vi "Test_OpenCloseTableRef_NoError.vi"(8 "error in (no error)":errorcluster, 11 "TestCase in":refnum<class "TestTopicLookupTable.lvclass">) -> (0 "error out":errorcluster, 3 "TestCase out":refnum<class "TestTopicLookupTable.lvclass">)   [LabVIEW 2017, in "TestTopicLookupTable.lvclass"]
uses:
  TestTopicLookupTable.lvclass
  Source/Mediator/TopicLookupTable/TopicLookupTable.lvclass
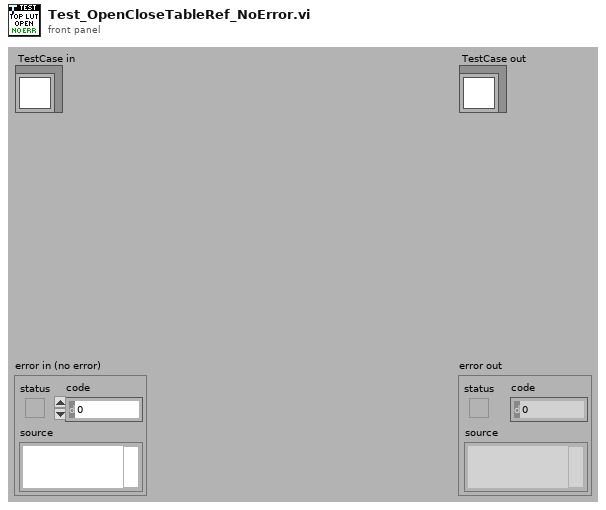
[diagram p1: front panel]
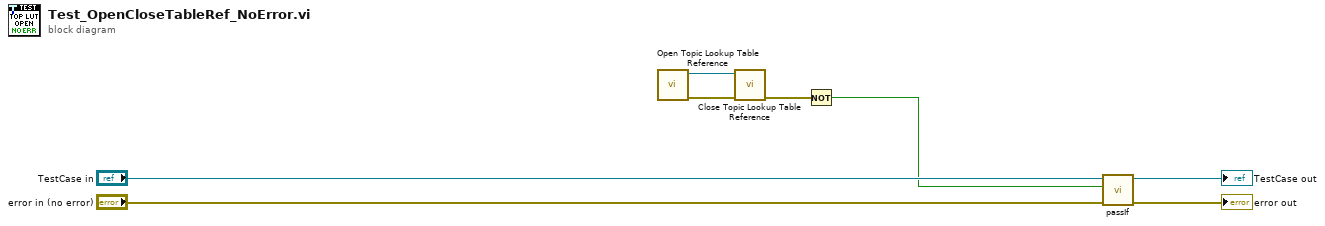
[diagram p0: block diagram]
diagram:
  n1 = call "Open Topic Lookup Table Reference.vi"() -> ("error out"=w4:errorcluster, "TopicLookupTable Reference"=w1:refnum<data-value>)  [unwired: 10 in]
  n2 = call "Close Topic Lookup Table Reference.vi"("error in (no error)"=w4, "TopicLookupTable"=w1) -> ("error out"=w2:errorcluster)  [unwired: 9 in]
  n3 = Not(x=w2) -> (.not. x?=w3:bool)
  n4 = call-dynamic "passIf.vi"("error in (no error)"="error in (no error)", "pass"=w3, "TestCase in"="TestCase in") -> ("error out"=→"error out":errorcluster, "TestCase out"=→"TestCase out":refnum<class "TestTopicLookupTable.lvclass">)  [unwired: 7 in]
